vi "B2G2_sqlite_createtable.vi"(8 "error in (no error)":errorcluster, 11 "Database File":string) -> (0 "error out":errorcluster)   [LabVIEW 2011]
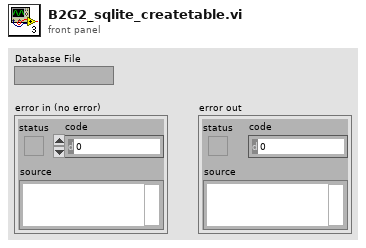
[diagram p1: front panel]
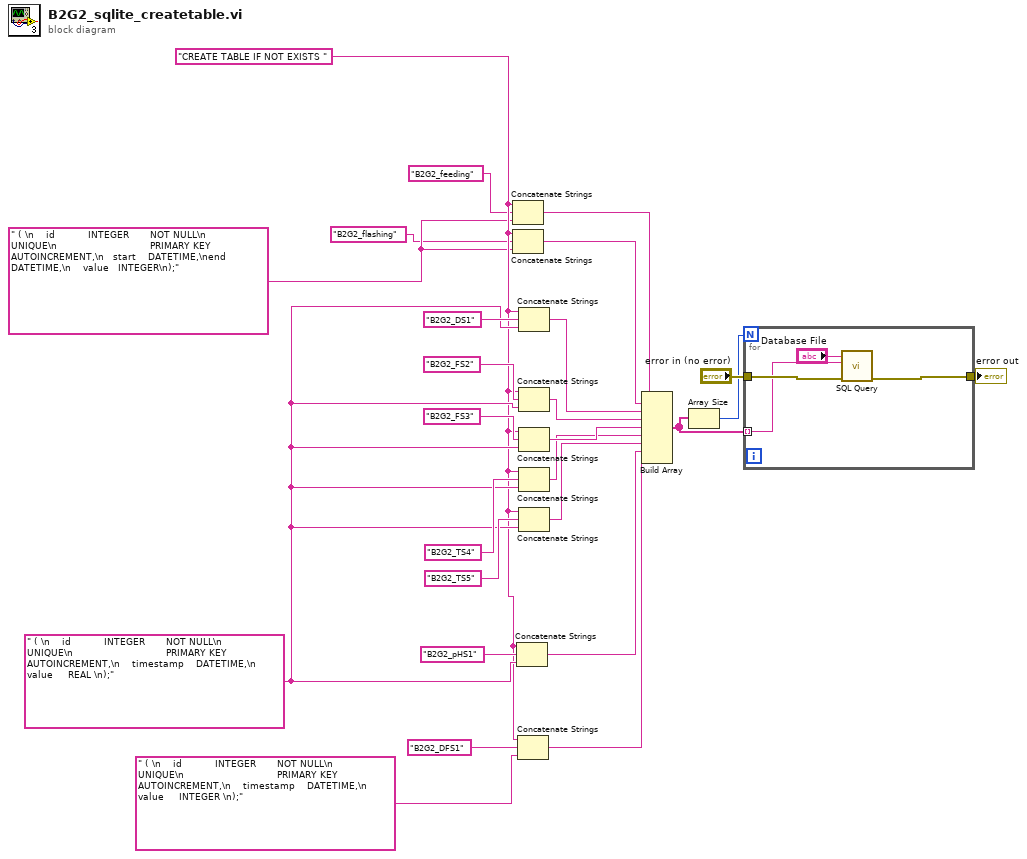
[diagram p0: block diagram]
diagram:
  w8 = " ( \n    id           INTEGER       NOT NULL\n                               UNIQUE\n                               PRIMARY KEY AUTOINCREMENT,\n    timestamp    DATETIME,\n    value     REAL \n);" ("SQL Query")
  w4 = "CREATE TABLE IF NOT EXISTS " ("SQL Query")
  w3 = " ( \n    id           INTEGER       NOT NULL\n                               UNIQUE\n                               PRIMARY KEY AUTOINCREMENT,\n   start    DATETIME,\nend    DATETIME,\n    value   INTEGER\n);" ("SQL Query")
  n1 = Concatenate Strings(w4, "B2G2_feeding" ("SQL Query"), w3) -> (w5:string)
  n2 = Concatenate Strings(w4, "B2G2_flashing" ("SQL Query"), w3) -> (w6:string)
  n3 = Concatenate Strings(w4, "B2G2_pHS1" ("SQL Query"), w8) -> (w9:string)
  n4 = Concatenate Strings(w4, "B2G2_DFS1" ("SQL Query"), " ( \n    id           INTEGER       NOT NULL\n                               UNIQUE\n                               PRIMARY KEY AUTOINCREMENT,\n    timestamp    DATETIME,\n    value     INTEGER \n);" ("SQL Query")) -> (w11:string)
  n5 = Concatenate Strings(w4, "B2G2_DS1" ("SQL Query"), w8) -> (w22:string)
  n6 = Concatenate Strings(w4, "B2G2_FS2" ("SQL Query"), w8) -> (w19:string)
  n7 = Concatenate Strings(w4, "B2G2_FS3" ("SQL Query"), w8) -> (w18:string)
  n8 = Concatenate Strings(w4, "B2G2_TS4" ("SQL Query"), w8) -> (w16:string)
  n9 = Concatenate Strings(w4, "B2G2_TS5" ("SQL Query"), w8) -> (w15:string)
  n10 = Build Array(w5, w6, w22, w19, w18, w16, w15, w9, w11) -> (w24:string[])
  n11 = Array Size(array=w24) -> (size(s)=w25:i32)
  n12 = for {
    N: w25 -> [_]
    tunnel: "error in (no error)" -> [w30]
    tunnel: w24 -> [w29] mode=indexing
    tunnel: [w28] -> w23
    n13 = call "SQL Query.vi"("error in (no error)"=w30, "SQL Query"=w29, "Database File"="Database File") -> ("error out"=w28:errorcluster)  [unwired: 6 in, 2 out]
  }
  "error out" <- w23
